vi "Stop Core.vi"(10 "final error code":i32, 11 "Bioreactor in":refnum<class "Bioreactor.lvclass">) -> (3 "Bioreactor out":refnum<class "Bioreactor.lvclass">)   [LabVIEW 2013, in "Bioreactor.lvlib" / "Bioreactor.lvclass"]
uses:
  Bioreactor.lvclass
  PluginInterface/PluginInterface.lvlibp/PluginInterfaceClass/PluginInterface.lvclass
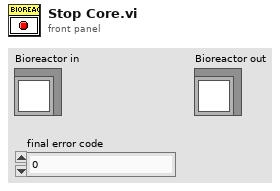
[diagram p1: front panel]
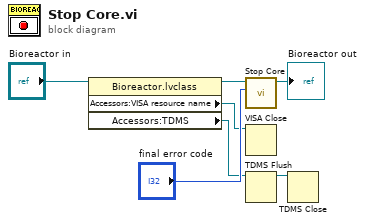
[diagram p0: block diagram]
diagram:
  n1 = property class="Bioreactor.lvclass"(reference="Bioreactor in") -> (reference out=w4:refnum<class "Bioreactor.lvclass">, "Accessors:VISA resource name"=w3:refnum<visa-resource-name>, "Accessors:TDMS"=w2:refnum<k34>)  [unwired: 1 in, 1 out]
  n2 = call-parent "Stop Core.vi"("final error code"="final error code", "Actor in"=w4) -> ("Actor out"=→"Bioreactor out":refnum<class "Bioreactor.lvclass">)  [unwired: 9 in]
  n3 = VISA Close(VISA resource name=w3) -> ()  [unwired: 1 in, 1 out]
  n4 = TDMS Flush(7:w2) -> (3:w1:refnum<k34>)  [unwired: 1 in, 1 out]
  n5 = TDMS Close(11:w1) -> ()  [unwired: 1 in, 2 out]
